vi "Read Item Tag.vi"(8 "error in (no error)":errorcluster, 11 "TreeItemCloseMsg in":refnum<class "TreeItemCloseMsg.lvclass">) -> (0 "error out":errorcluster, 2 "Item Tag":string, 3 "TreeItemCloseMsg out":refnum<class "TreeItemCloseMsg.lvclass">)   [LabVIEW 2020, in "ActorEvents.lvlib" / "TreeItemCloseMsg.lvclass"]
uses:
  <vilib>/gpm_packages/@cs/mva-viewable/Source/ActorEvents/IEventAggregator Messages/TreeItemCloseMsg/TreeItemCloseMsg.lvclass
  <vilib>/gpm_packages/@cs/mva-viewable/Source/ActorEvents/IEventAggregator Messages/TreeItemCloseMsg/TreeItemCloseMsg.lvclass/TreeItemCloseMsg.ctl
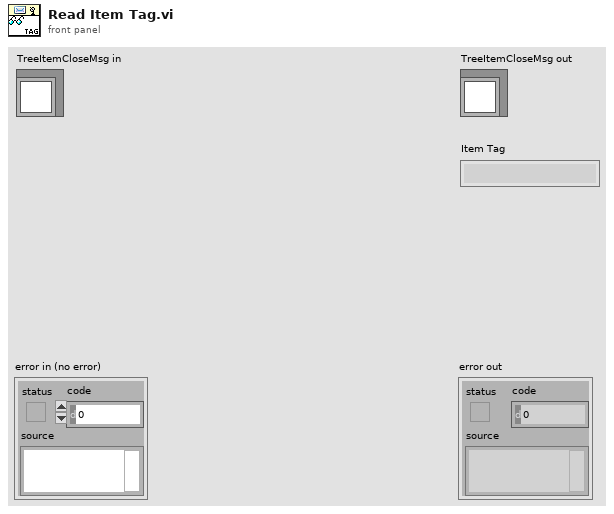
[diagram p1: front panel]
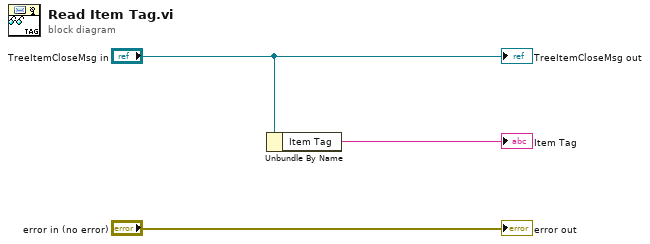
[diagram p0: block diagram]
diagram:
  n1 = Unbundle By Name("TreeItemCloseMsg in") -> ("Item Tag"=→"Item Tag":string)
  "error out" <- "error in (no error)"
  "TreeItemCloseMsg out" <- "TreeItemCloseMsg in"
